vi "Read Driver Joystick.vi"(11 "Driver Joystick":T1) -> ()   [LabVIEW 2019]
uses:
  <vilib>/Rock Robotics/WPI/Joystick/WPI_JoystickDevRef.ctl
  <vilib>/Rock Robotics/WPI/Joystick/WPI_JoystickDeviceEnum.ctl
  Framework/Robot Global Data.vi
panel:
  # "READ DRIVER JOYSTICK"
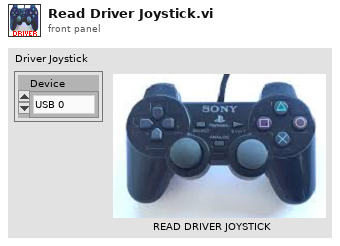
[diagram p1: front panel]
types:
  T1 = typedef "WPI_JoystickDevRef.ctl" = cluster{"Device":T2}
  T2 = typedef "WPI_JoystickDeviceEnum.ctl" = enum16{"USB 0", "USB 1", "USB 2", "USB 3", "USB 4", "USB 5"}
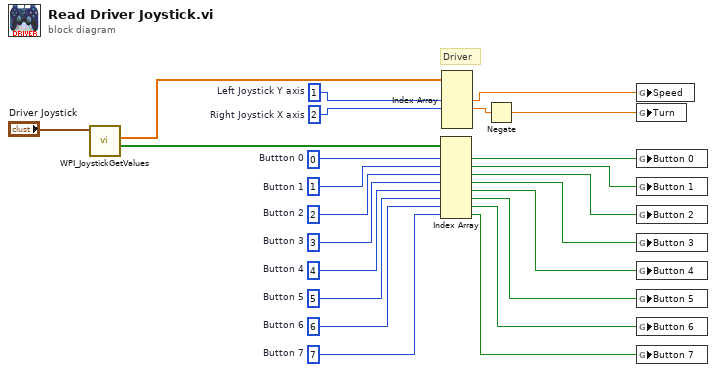
[diagram p0: block diagram]
diagram:
  w7 = 7  # Button 7
  w19 = 6  # Button 6
  w18 = 5  # Button 5
  w20 = 4  # Button 4
  w21 = 3  # Button 3
  w22 = 2  # Button 2
  w23 = 1  # Button 1
  w24 = 0  # Buttton 0
  w1 = 2  # Right Joystick X axis
  w2 = 1  # Left Joystick Y axis
  # "Driver"
  n1 = call <vilib>:"WPI_JoystickGetValues.vi"("JoystickDevRef"="Driver Joystick") -> ("Buttons"=w16:bool[], "Axes"=w15:dbl[])  [unwired: 6 in, 3 out]
  n2 = Index Array(array=w16, index #1=w24, index #2=w23, index #3=w22, index #4=w21, index #5=w20, index #6=w18, index #7=w19, index #8=w7) -> (element #1=w17:bool, element #2=w14:bool, element #3=w13:bool, element #4=w9:bool, element #5=w12:bool, element #6=w11:bool, element #7=w10:bool, element #8=w8:bool)
  n3 = Index Array(array=w15, index #2=w2, index #3=w1) -> (element #2=w3:dbl, element #3=w4:dbl)  [unwired: 3 in, 3 out]
  n4 = Negate(x=w4) -> (-x=w6:dbl)
  n5 = global write "Robot Global Data.vi" "Speed"(w3) -> ()
  n6 = global write "Robot Global Data.vi" "Turn"(w6) -> ()
  n7 = global write "Robot Global Data.vi" "Button 0"(w17) -> ()
  n8 = global write "Robot Global Data.vi" "Button 1"(w14) -> ()
  n9 = global write "Robot Global Data.vi" "Button 2"(w13) -> ()
  n10 = global write "Robot Global Data.vi" "Button 3"(w9) -> ()
  n11 = global write "Robot Global Data.vi" "Button 4"(w12) -> ()
  n12 = global write "Robot Global Data.vi" "Button 5"(w11) -> ()
  n13 = global write "Robot Global Data.vi" "Button 6"(w10) -> ()
  n14 = global write "Robot Global Data.vi" "Button 7"(w8) -> ()
